vi "level motor control.vi"() -> ()   [LabVIEW 2019]
uses:
  <vilib>/MakerHub/LINX/Public/Peripherals/Digital/Digital Write 1 Chan.vi
  <vilib>/MakerHub/LINX/Public/Peripherals/PWM/PWM Set Duty Cycle 1 Chan.vi
  <vilib>/MakerHub/LINX/Public/Peripherals/Digital/Digital Write N Chans.vi
  <vilib>/MakerHub/LINX/Private/Local IO/LinxDigitalWrite.vi
  <vilib>/MakerHub/LINX/Public/Utilities/Check Channel.vi
  <vilib>/MakerHub/LINX/Public/Utilities/Open Serial.vi
  <vilib>/MakerHub/LINX/Private/Utilties/Generate Error.vi
  <vilib>/MakerHub/LINX/Public/Peripherals/PWM/PWM Set Duty Cycle N Chans.vi
  <vilib>/MakerHub/LINX/LMH-LINX.lvlib
panel:
  in  "y 3":dbl
  in  "y 2":dbl
  in  "y":dbl
  in  "Slide":dbl(slide) scale=0.0..10.0
  in  "Serial Port":refnum<visa-resource-name>="N/A"
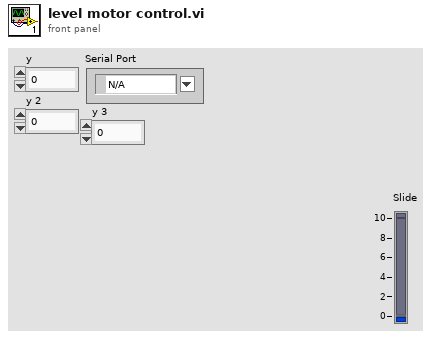
[diagram p1: front panel]
types:
  T1 = typedef "LMH-LINX.lvlib/LINX Ref.ctl" = cluster{"IO":T2, "Interface":T3, "LINX Device Config":T4}
  T2 = typedef "LMH-LINX.lvlib/Platform.ctl" = enum16{"Remote", "Local"}
  T3 = typedef "LMH-LINX.lvlib/Interface.ctl" = enum16{"Serial", "TCP"}
  T4 = typedef "LMH-LINX.lvlib/Device.lvlib/LINX Device Config.ctl" = cluster{"Interface":T3, "COM Port":refnum<visa-resource-name>, "TCP Configuration":T5, "Device Family":u8, "Device ID":u8, "Device Name":string, "TCP Ref":refnum<k5>, "Channels":T6}
  T5 = typedef "LMH-LINX.lvlib/Device.lvlib/TCP Config.ctl" = cluster{"IP Address":string, "Port":u16}
  T6 = typedef "LMH-LINX.lvlib/Channels.ctl" = cluster{"DI":u8[], "DO":u8[], "AI":u8[], "AO":u8[], "PWM":u8[], "QE":u8[], "UART":u8[], "I2C 2":u8[], "SPI":u8[], "CAN":u8[], "Servo":u8[], "AI Ref (V)":dbl, "AI Resolution (Bits)":u8, "AO Ref (V)":dbl, "AO Resolution (Bits)":u8}
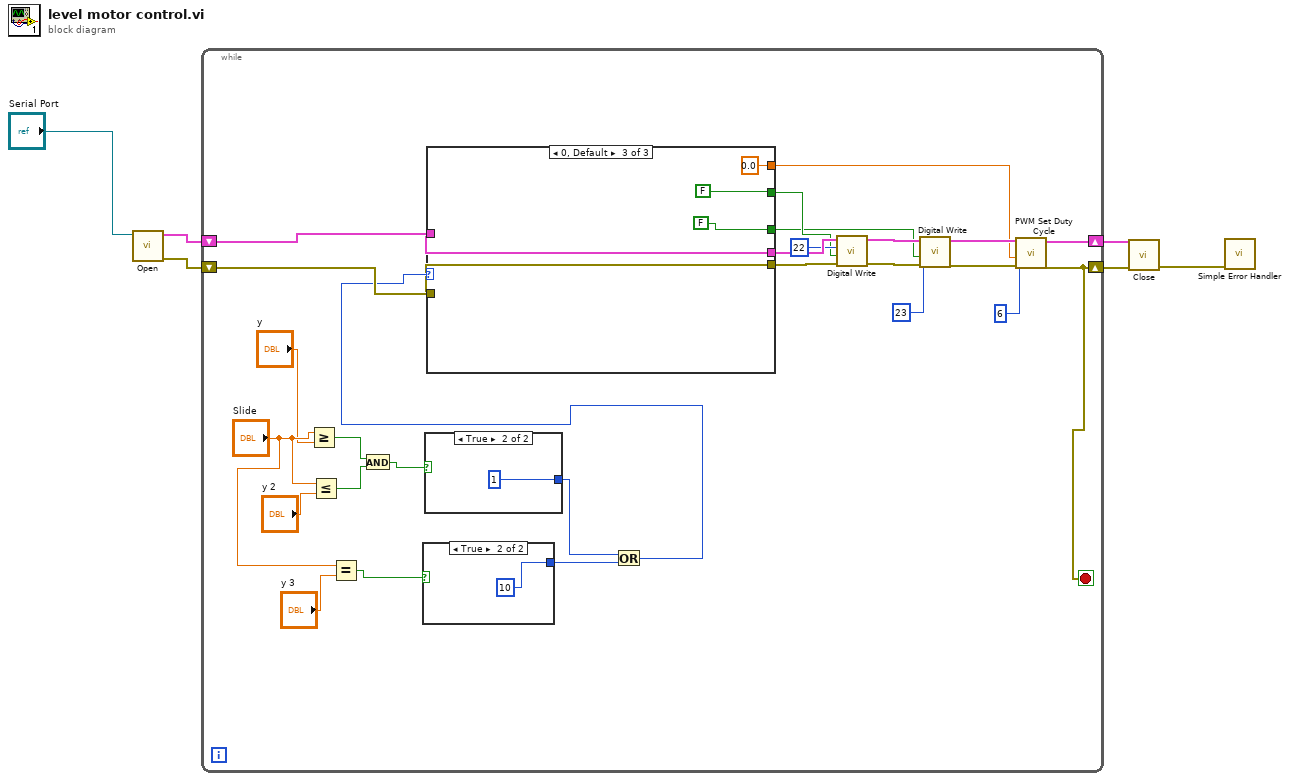
[diagram p0: block diagram]
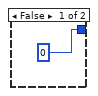
[diagram p2: hidden frame]
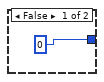
[diagram p3: hidden frame]
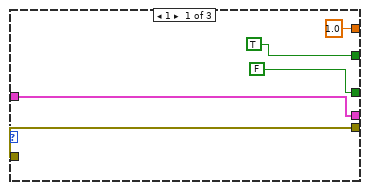
[diagram p4: hidden frame]
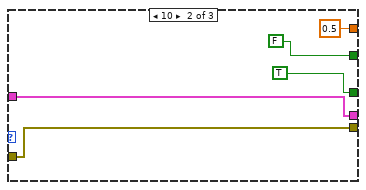
[diagram p5: hidden frame]
diagram:
  n1 = call-poly <vilib>:"Open.vi"("Serial Port"="Serial Port") -> ("Error Out"=w3:errorcluster, "LINX Resource"=w6:T1)  [unwired: 8 in, 1 out]
  n2 = while {
    shift-right: [w29] -> w5
    shift-left: w6 -> [w32]
    shift-right: [w18] -> w4
    shift-left: w3 -> [w26]
    stop <- w18 stop-if-true
    n3 = Greater Or Equal?(x="Slide", y="y") -> (x >= y?=w17:bool)
    n4 = Less Or Equal?(x="Slide", y="y 2") -> (x <= y?=w16:bool)
    n5 = Equal?(x="Slide", y="y 3") -> (x = y?=w13:bool)
    n6 = And(x=w17, y=w16) -> (x .and. y?=w15:bool)
    n7 = case shown="True" w13 {
      tunnel: [0 10] -> w11
      frame False {
      }
      frame True {
      }
    }
    n8 = case shown="True" w15 {
      tunnel: [0 1] -> w12
      frame False {
      }
      frame True {
      }
    }
    n9 = Or(x=w12, y=w11) -> (x .or. y?=w10:i32)
    n10 = case shown="0, Default" w10 {
      tunnel: [w42 w47 w52] -> w33
      tunnel: w32 -> [w42 w47 w52]
      tunnel: w26 -> [w41 w46 w51]
      tunnel: [w41 w46 w51] -> w25
      tunnel: [TRUE FALSE FALSE] -> w21
      tunnel: [FALSE TRUE FALSE] -> w20
      tunnel: [1.0 ("Duty Cycle (0-1)") 0.5 ("Duty Cycle (0-1)") 0.0 ("Duty Cycle (0-1)")] -> w19
      frame 1 {
      }
      frame 10 {
      }
      frame 0, Default {
      }
    }
    n11 = call-poly <vilib>:"Digital Write.vi"("Error In"=w25, "Output Value"=w21, "DO Channel"=u8 22, "LINX Resource"=w33) -> ("Error Out"=w27:errorcluster, "LINX Resource"=w31:T1)  [unwired: 6 in]
    n12 = call-poly <vilib>:"Digital Write.vi"("Error In"=w27, "Output Value"=w20, "DO Channel"=u8 23, "LINX Resource"=w31) -> ("Error Out"=w28:errorcluster, "LINX Resource"=w30:T1)  [unwired: 6 in]
    n13 = call-poly <vilib>:"PWM Set Duty Cycle.vi"("Error In"=w28, "Duty Cycle (0-1)"=w19, "PWM Channel"=u8 6, "LINX Resource"=w30) -> ("Error Out"=w18:errorcluster, "LINX Resource"=w29:T1)  [unwired: 6 in]
  }
  n14 = call <vilib>:"Close.vi"("Error In"=w4, "LINX Resource"=w5) -> ("Error Out"=w1:errorcluster)  [unwired: 9 in]
  n15 = call <vilib>:"Simple Error Handler.vi"("error in (no error)"=w1) -> ()  [unwired: 4 in, 5 out]
